vi "checkout.vi"(7 "locked by?":string, 8 "error in (no error)":errorcluster) -> (0 "error out":errorcluster, 3 "GenericScanMode out":refnum<class "GenericImagingMode.lvclass">)   [LabVIEW 2010, in "GenericImagingMode.lvclass"]
uses:
  GenericImagingMode.lvclass
  class_data.vi
  common/classes/ErrorController/ErrorController/class_data.vi
  common/classes/GenericComponent/GenericComponent/GenericComponent.lvclass
  common/classes/ErrorController/ErrorController/ErrorController.lvclass
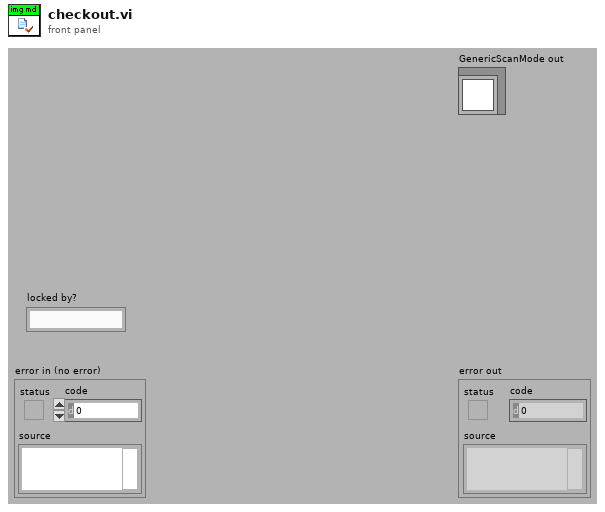
[diagram p1: front panel]
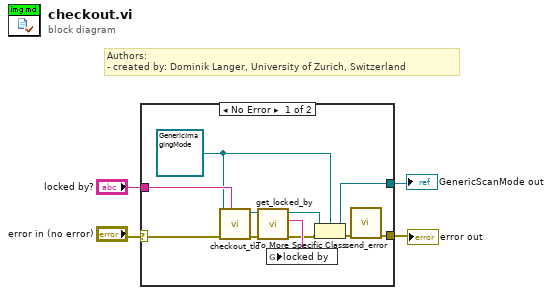
[diagram p0: block diagram]
diagram:
  # "Authors: \n- created by: Dominik Langer, University of Zurich, Switzerland"
  n1 = case shown="No Error" "error in (no error)" {
    selector: "error in (no error)" -> [w8 w16]
    tunnel: [w6 w16] -> w4
    tunnel: "locked by?" -> [w15 _]
    tunnel: [w14 _] -> w1
    frame No Error {
      w5 = refnum<class "GenericImagingMode.lvclass"> refnum ("GenericScanMode.lvclass")
      n2 = call-dynamic "checkout_tlc.vi"("locked by?"=w15, "error in (no error)"=w8, "GenericToplevelComponent in"=w5) -> ("error out"=w13:errorcluster, "GenericToplevelComponent out"=w12:refnum<class "GenericToplevelComponent.lvclass">)  [unwired: 7 in]
      n3 = call "get_locked_by.vi"("error in (no error)"=w13, "GenericPlugin.lvclass in"=w12) -> ("error out"=w10:errorcluster, "locked by"=w11:string, "GenericPlugin.lvclass out"=w9:refnum<class "GenericToplevelComponent.lvclass">)  [unwired: 7 out]
      n4 = global write "class_data.vi" "locked by"(w11) -> ()
      n5 = To More Specific Class(target class=w5, reference=w9, error in=w10) -> (specific class reference=w14:refnum<class "GenericImagingMode.lvclass">, error out=w7:errorcluster)
      n6 = call "send_error.vi"("error in (no error)"=w7) -> ("error out"=w6:errorcluster)  [unwired: 10 in]
    }
    frame Error {
    }
  }
  "error out" <- w4
  "GenericScanMode out" <- w1
